vi "get registration.vi"(8 "error in":errorcluster, 11 "event reporter in":refnum<class "event reporter.lvclass">) -> (0 "error out":errorcluster, 2 "result registration":refnum<event-registration>, 3 "event reporter out":refnum<class "event reporter.lvclass">)   [LabVIEW 2013, in "event reporter.lvclass"]
uses:
  event reporter.lvclass
  result/result.lvclass
  event reporter.lvclass/event reporter.ctl
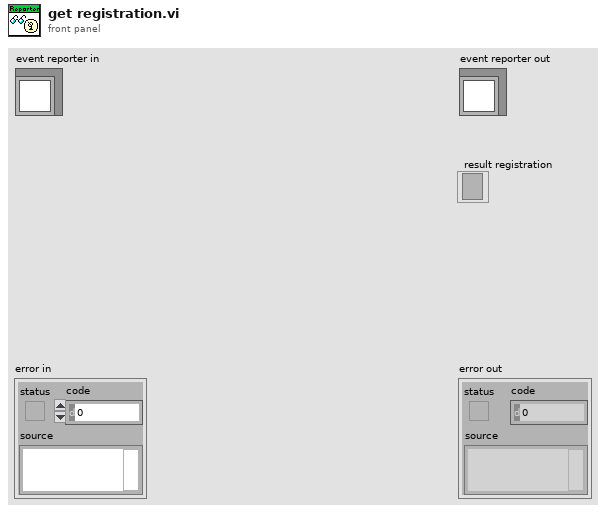
[diagram p1: front panel]
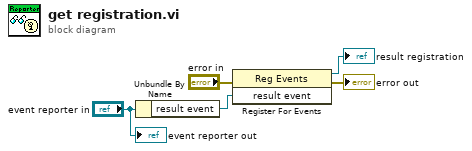
[diagram p0: block diagram]
diagram:
  n1 = Unbundle By Name("event reporter in") -> ("result event"=w2:refnum<user-event>)
  n2 = register-events(error in="error in", w2) -> (reference out=→"result registration":refnum<event-registration>, error out=→"error out":errorcluster)  [unwired: 1 in]
  "event reporter out" <- "event reporter in"
